vi "Temperature Warnings.vi"() -> ()   [LabVIEW 2021]
doc: "This VI is used to determine the string to output to the weather station based on the current temperature and limit settings.\n\nInputs: Current Temperature (DBL), Minimum Temperature (DBL), and Maximum Temperature (DBL).\nOutputs: Warning Text (string) and Warning? (Boolean)."
panel:
  out "Weather Data Out":T1={"Current Temperature"=0.0, "Max Temperature"=0.0, "Min Temperature"=0.0, "Warning?"=FALSE, "Warning Text"="No Warning"}
  in  "Weather Data In":T1={"Current Temperature"=0.0, "Max Temperature"=0.0, "Min Temperature"=0.0, "Warning?"=FALSE, "Warning Text"="No Warning"}
  out "Error Out":errorcluster
  in  "Error In":errorcluster
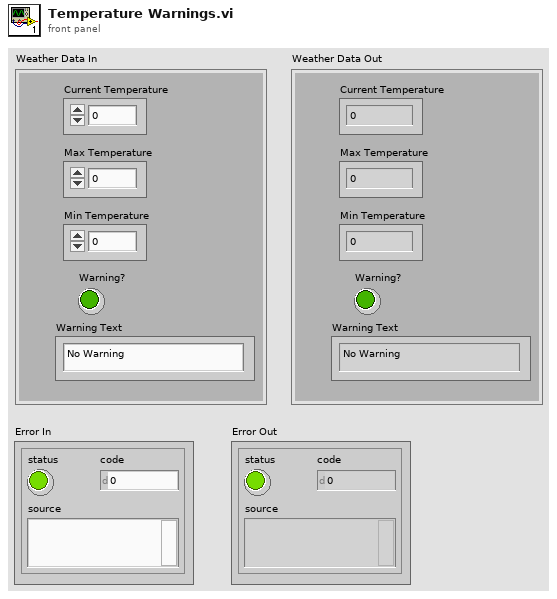
[diagram p1: front panel]
types:
  T1 = typedef "WeatherData.ctl" = cluster{"Current Temperature":dbl, "Max Temperature":dbl, "Min Temperature":dbl, "Warning?":bool, "Warning Text":string}
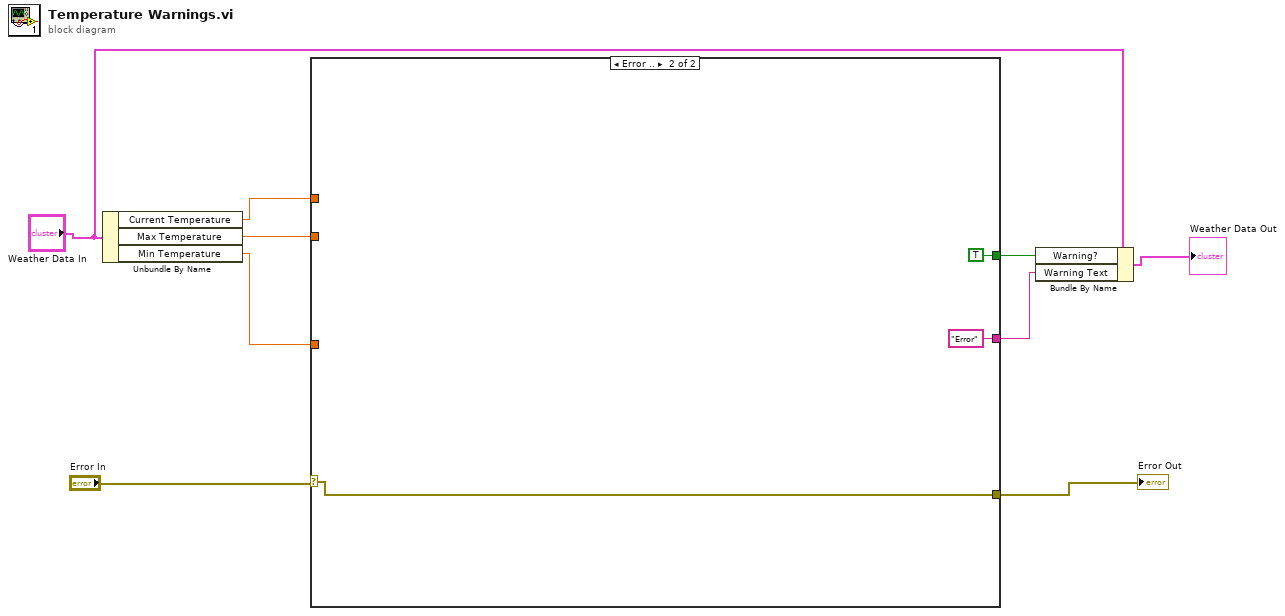
[diagram p0: block diagram]
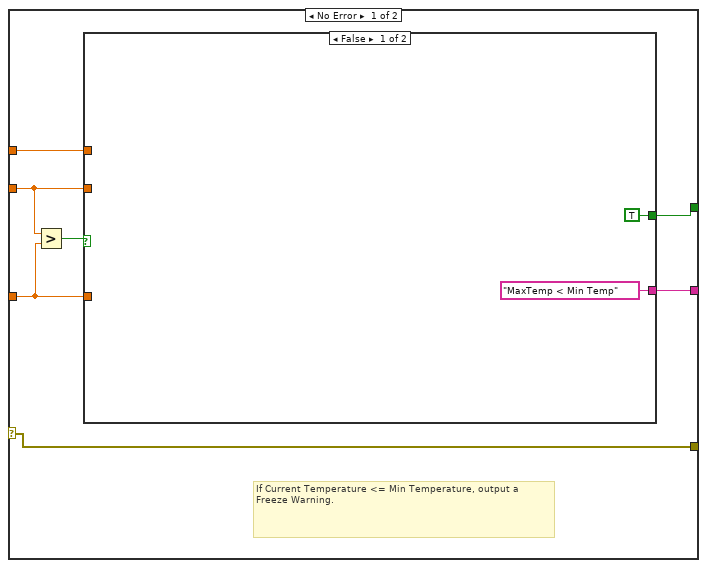
[diagram p2: hidden frame]
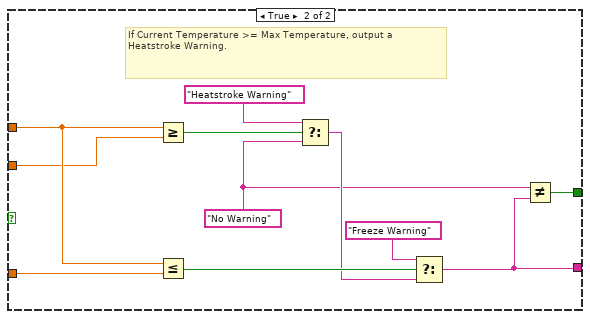
[diagram p3: hidden frame]
diagram:
  n1 = Unbundle By Name("Weather Data In") -> ("Current Temperature"=w9:dbl, "Max Temperature"=w8:dbl, "Min Temperature"=w7:dbl)
  n2 = case shown="Error .." "Error In" {
    selector: "Error In" -> [w13 w32]
    tunnel: w9 -> [w16 _]
    tunnel: w8 -> [w11 _]
    tunnel: w7 -> [w10 _]
    tunnel: [w15 TRUE] -> w5
    tunnel: [w14 "Error" ("f")] -> w4
    tunnel: [w13 w32] -> w1
    frame No Error {
      # "If Current Temperature <= Min Temperature, output a Freeze Warning."
      n3 = Greater?(x=w11, y=w10) -> (0:w12:bool)
      n4 = case shown="False" w12 {
        tunnel: w16 -> [_ w23]
        tunnel: w11 -> [_ w22]
        tunnel: w10 -> [_ w21]
        tunnel: [TRUE w20] -> w15
        tunnel: ["MaxTemp < Min Temp" ("f") w19] -> w14
        frame False {
        }
        frame True {
          w24 = "No Warning" ("f")
          # "If Current Temperature >= Max Temperature, output a Heatstroke Warning."
          n5 = Greater Or Equal?(x=w23, y=w22) -> (x >= y?=w29:bool)
          n6 = Less Or Equal?(x=w23, y=w21) -> (x <= y?=w26:bool)
          n7 = Select(t="Heatstroke Warning", s=w29, f=w24) -> (s? t:f=w25:string)
          n8 = Select(t="Freeze Warning", s=w26, f=w25) -> (s? t:f=w19:string)
          n9 = Not Equal?(x=w24, y=w19) -> (x != y?=w20:bool)
        }
      }
    }
    frame Error {
    }
  }
  "Error Out" <- w1
  n10 = Bundle By Name(cluster="Weather Data In", "Warning?"=w5, "Warning Text"=w4) -> (→"Weather Data Out":T1)
